vi "testStageTriggering.vi"() -> ()   [LabVIEW 2015]
panel:
  in  "initTrigPos (mm)":dbl=0.5
  out "error out":errorcluster
  in  "motionSelection":enum32{"stop/ start", "cont."}(radio)=enum."cont."
  in  "stepSize (mm)":dbl=0.5
  in  "finPos (mm)":dbl=10.0
  in  "initPos (mm)":dbl=5.0
  in  "triggOutputIdx":string="3"
  in  "System no.":i32=2 min=1 step=1
  in  "zIdx":i32=1
  in  "error in":errorcluster
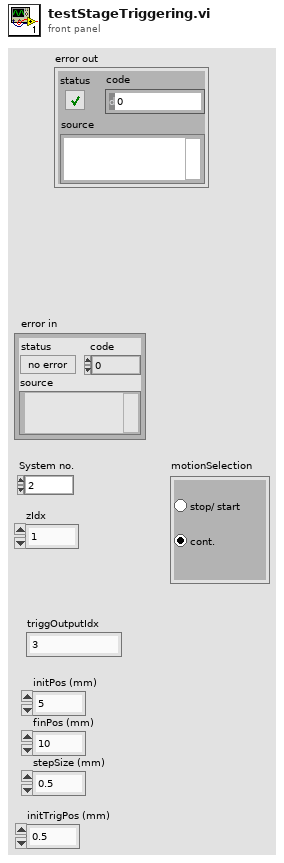
[diagram p1: front panel]
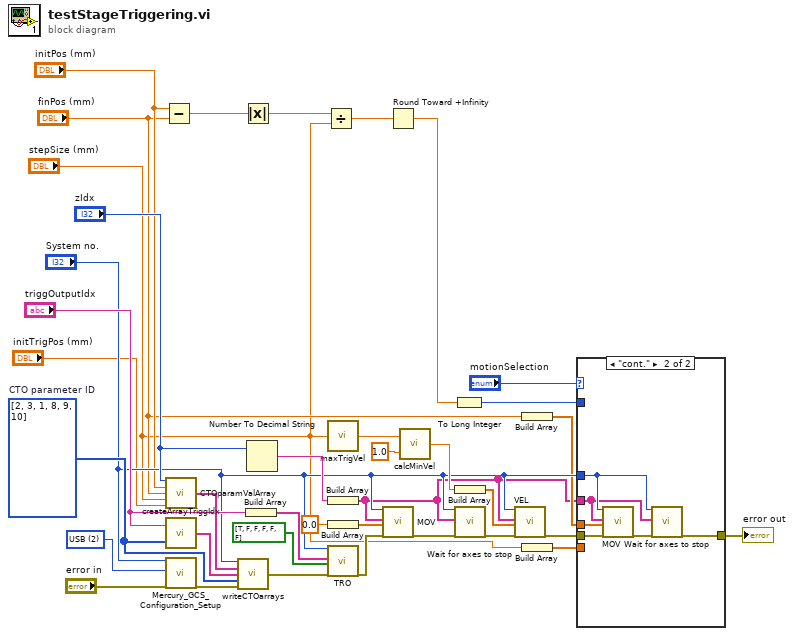
[diagram p0: block diagram]
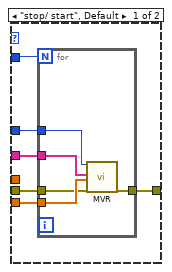
[diagram p2: hidden frame]
diagram:
  w34 = i32[] [2, 3, 1, 8, 9, 10]  # CTO parameter ID
  w36 = u16 2 items=["RS232", "RS232 DaisyChain", "USB", "USB_DaisyChain"] ("Interface")
  n1 = Subtract(x="initPos (mm)", y="finPos (mm)") -> (x-y=w11:dbl)
  n2 = call "CTOparamValArray.vi"("zIdx"="zIdx", "initPos (mm)"="initPos (mm)", "finPos (mm)"="finPos (mm)", "stepSize (mm)"="stepSize (mm)", "initTrigPos (mm)"="initTrigPos (mm)") -> ("CTOparamValArray"=w33:string[])  [unwired: 10 in]
  n3 = call "createArrayTriggIdx.vi"("CTO parameter ID"=w34, "triggOutputIdx"="triggOutputIdx") -> ("Array"=w35:string[])
  n4 = call "Mercury_GCS_Configuration_Setup.vi"("System no."="System no.", "Interface"=w36, "error in"="error in") -> ("error out"=w32:errorcluster)  [unwired: 10 in, 6 out]
  n5 = call "writeCTOarrays.vi"("System no."="System no.", "CTOparamValArray"=w33, "triggIdxArray"=w35, "CTO parameter ID"=w34, "error in"=w32) -> ("error out"=w31:errorcluster)  [unwired: 10 in]
  n6 = Absolute Value(x=w11) -> (abs(x)=w10:dbl)
  n7 = Build Array("triggOutputIdx") -> (w29:string[])
  n8 = Number To Decimal String(number="zIdx") -> (decimal integer string=w24:string)  [unwired: 1 in]
  n9 = Divide(x=w10, y="stepSize (mm)") -> (x/y=w9:dbl)
  n10 = call "maxTrigVel.vi"("stepSize (mm)"="stepSize (mm)") -> ("maxVel (mm/s)"=w23:dbl)
  n11 = Build Array(w24) -> (w5:string[])
  n12 = Build Array(0.0 ("element")) -> (w1:dbl[])
  n13 = call "TRO.vi"("System no."="System no.", "TriggerOut to command"=w29, "Trigger status"=bool[] [TRUE, FALSE, FALSE, FALSE, FALSE, FALSE], "error in"=w31) -> ("error out"=w26:errorcluster)  [unwired: 15 in]
  n14 = call "MOV.vi"("System no."="System no.", "Axes to move"=w5, "Position values"=w1, "error in"=w26) -> ("error out"=w27:errorcluster)  [unwired: 15 in]
  n15 = Round Toward +Infinity(x=w9) -> (ceil(x): smallest int >= x=w14:dbl)
  n16 = call "calcMinVel.vi"("velocity2"=1.0, "velocity1"=w23) -> ("minVal"=w21:dbl)
  n17 = To Long Integer(number=w14) -> (32bit integer=w8:i32)
  n18 = Build Array(w21) -> (w20:dbl[])
  n19 = call "Wait for axes to stop.vi"("System no."="System no.", "Axes to wait for"=w5, "error in"=w27) -> ("error out"=w19:errorcluster)  [unwired: 4 in, 12 out]
  n20 = call "VEL.vi"("System no."="System no.", "Axes to set"=w5, "Velocity values"=w20, "error in"=w19) -> ("error out"=w15:errorcluster)  [unwired: 14 in, 1 out]
  n21 = Build Array("finPos (mm)") -> (w16:dbl[])
  n22 = Build Array("stepSize (mm)") -> (w6:dbl[])
  n23 = case shown="\"cont.\"" "motionSelection" {
    tunnel: "System no." -> [w42 w51]
    tunnel: w5 -> [w41 w50]
    tunnel: w16 -> [_ w54]
    tunnel: w15 -> [w39 w53]
    tunnel: [w38 w49] -> w4
    tunnel: w8 -> [w43 _]
    tunnel: w6 -> [w40 _]
    frame "stop/ start", Default {
      n24 = for {
        N: w43 -> [_]
        tunnel: w42 -> [w48]
        tunnel: w41 -> [w47]
        tunnel: w40 -> [w46]
        tunnel: w39 -> [w45]
        tunnel: [w44] -> w38
        n25 = call "MVR.vi"("System no."=w48, "Axes to move"=w47, "Position values"=w46, "error in"=w45) -> ("error out"=w44:errorcluster)  [unwired: 1 in, 14 out]
      }
    }
    frame "cont." {
      n26 = call "MOV.vi"("System no."=w51, "Axes to move"=w50, "Position values"=w54, "error in"=w53) -> ("error out"=w52:errorcluster)  [unwired: 15 in]
      n27 = call "Wait for axes to stop.vi"("System no."=w51, "Axes to wait for"=w50, "error in"=w52) -> ("error out"=w49:errorcluster)  [unwired: 4 in, 12 out]
    }
  }
  "error out" <- w4
